vi "Alp Seq Alloc.vi"(7 "SequenceIdPtr":u32, 8 "error in (no error)":errorcluster, 9 "PicNum":i32, 10 "BitPlanes":i32, 11 "DeviceId":u32) -> (0 "error out":errorcluster, 3 "function return":i32, 5 "SequenceIdPtr out":u32)   [LabVIEW 2013, in "alpD41.lvlib"]
uses:
  alpD41.lvlib
  alpD41.dll
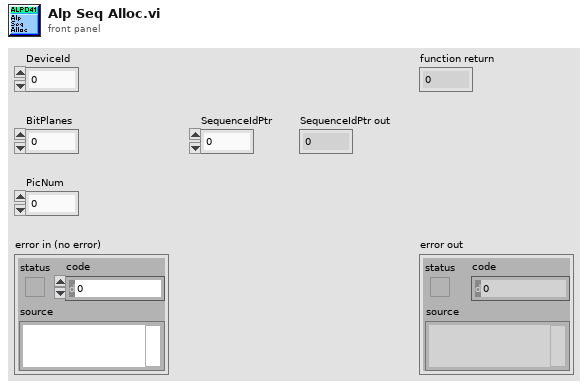
[diagram p1: front panel]
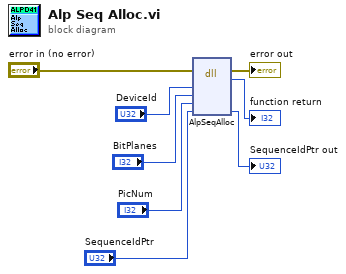
[diagram p0: block diagram]
diagram:
  n1 = dll-call lib="C:/Users/ErNa/Google Drive (ernajqi@gmail.com)/ErNa/LabView/DMD Standalone Codes/Libraries-alpD41/alpD41.*" fn="AlpSeqAlloc"(error in="error in (no error)", "DeviceId"="DeviceId", "BitPlanes"="BitPlanes", "PicNum"="PicNum", "SequenceIdPtr"="SequenceIdPtr") -> (error out=→"error out":errorcluster, →"function return":i32, "SequenceIdPtr"=→"SequenceIdPtr out":u32)  [unwired: 5 in, 1 out]
